vi "Intake Stay Open.vi"() -> (3 "Open?":bool)   [LabVIEW 2017]
uses:
  Robot Global Data.vi
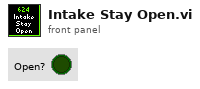
[diagram p1: front panel]
types:
  T1 = typedef "Intake Command Cluster.ctl" = cluster{"Intake Mode":T2, "Intake States":T3, "Manual Roller Power":dbl, "Manual Close?":bool, "Manual Lift Power":dbl, "Override Lift?":bool, "Override Angle":dbl}
  T2 = typedef "Intake Mode.ctl" = enum16{"Auto", "Semi Auto", "Manual"}
  T3 = typedef "Intake States.ctl" = enum16{"Zero", "Override Angle", "Idle", "Drop Mid", "Drop Low", "Outtake", "Intake"}
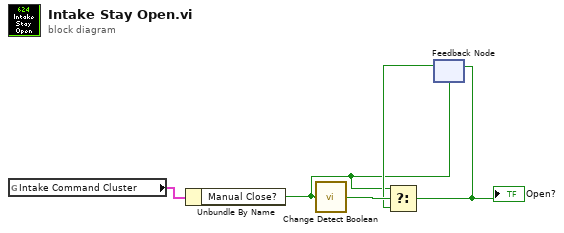
[diagram p0: block diagram]
diagram:
  n1 = global read "Robot Global Data.vi" "Intake Command Cluster"() -> (w5:T1)
  n2 = Unbundle By Name(w5) -> ("Manual Close?"=w2:bool)
  n3 = call "Change Detect Boolean.vi"("In"=w2) -> ("Changed?"=w4:bool)
  n4 = feedback #1(w2) -> (w3:bool)
  n5 = Select(t=w2, s=w4, f=w3) -> (s? t:f=w1:bool)
  "Open?" <- w1
  n6 = feedback-in #1(w1) -> ()
